vi "Write Observer Directory.vi"(10 "Observer Directory":string, 11 "ModuleConfigs in":refnum<class "ModuleConfigs.lvclass">) -> (3 "ModuleConfigs out":refnum<class "ModuleConfigs.lvclass">)   [LabVIEW 2014, in "ModuleConfigs.lvclass"]
uses:
  ModuleConfigs.lvclass
  ModuleConfigs.lvclass/ModuleConfigs.ctl
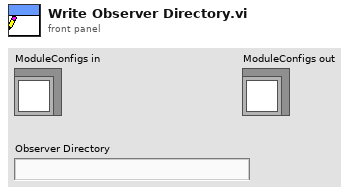
[diagram p1: front panel]
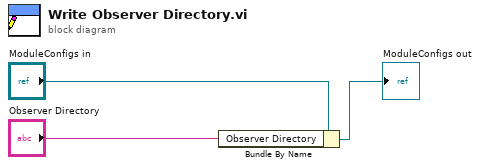
[diagram p0: block diagram]
diagram:
  n1 = Bundle By Name(cluster="ModuleConfigs in", "Observer Directory"="Observer Directory") -> (→"ModuleConfigs out":refnum<class "ModuleConfigs.lvclass">)
